vi "MeasurementServer_FourProbeMeasurementComplete.vi"(0 "gRPCid":T1, 3 "error in (no error)":errorcluster) -> (10 "error out":errorcluster)   [LabVIEW 2019]
uses:
  MeasurementServer_gRPCid.ctl
  build/Release/labview_measurement_server.dll
  labview-grpc-measurement-server.lvlib
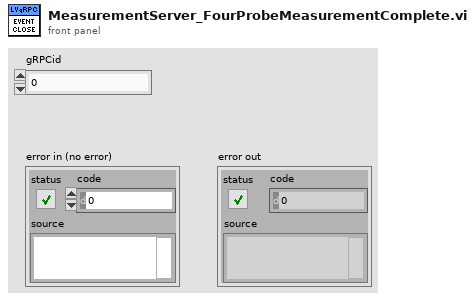
[diagram p1: front panel]
types:
  T1 = typedef "labview-grpc-measurement-server.lvlib/MeasurementServer_gRPCid.ctl" = u64
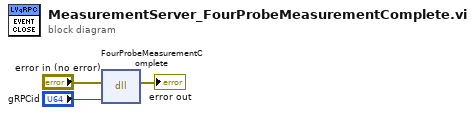
[diagram p0: block diagram]
diagram:
  n1 = dll-call lib="C:/Users/chericks/Desktop/OCV/labview-grpc-query-server/build/Release/labview_measurement_server.dll" fn="FourProbeMeasurementComplete"(error in="error in (no error)", "id"="gRPCid") -> (error out=→"error out":errorcluster)  [unwired: 4 in, 1 out]
